vi "Supply_ZeroCheck.vi"(8 "error in (no error)":errorcluster, 10 "enable/disable":bool, 11 "KE487 in":refnum<class "KE487.lvclass">) -> (0 "error out":errorcluster, 3 "KE487 out":refnum<class "KE487.lvclass">)   [LabVIEW 2018, in "KE487.lvclass"]
uses:
  KE487.lvclass
  C:/ProbeTestSoftware2019/itk-strip-sensor-qc/InstrControl/InstrControl.lvclass
  InstrControl.lvclass
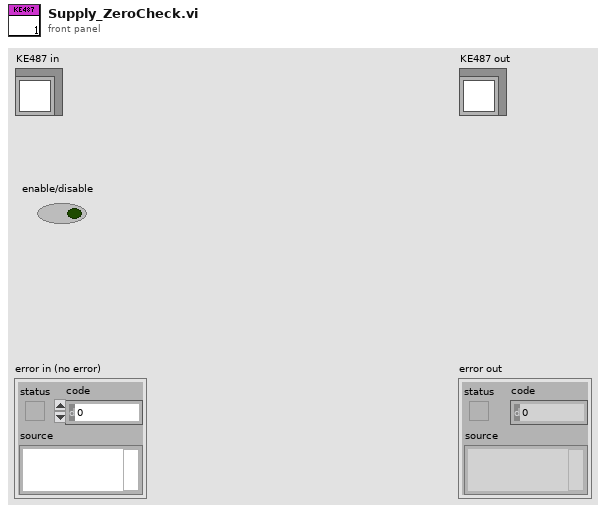
[diagram p1: front panel]
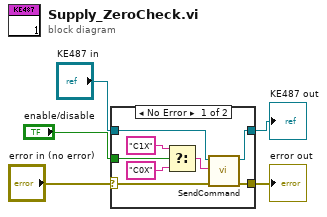
[diagram p0: block diagram]
diagram:
  n1 = case shown="No Error" "error in (no error)" {
    selector: "error in (no error)" -> [w11 w15]
    tunnel: [w10 w15] -> w4
    tunnel: [w12 w14] -> w2
    tunnel: "KE487 in" -> [w13 w14]
    tunnel: "enable/disable" -> [w9 _]
    frame No Error {
      n2 = Select(t="C1X", s=w9, f="C0X") -> (s? t:f=w6:string)
      n3 = call "SendCommand.vi"("error in (no error)"=w11, "Command string"=w6, "InstControl in"=w13) -> ("error out"=w10:errorcluster, "InstControl out"=w12:refnum<class "KE487.lvclass">)  [unwired: 7 in]
    }
    frame Error {
    }
  }
  "error out" <- w4
  "KE487 out" <- w2
